vi "Summary.vi"() -> ()   [LabVIEW 2017]
uses:
  d1a68c5a-fde4-43d3-b03d-75d6c03e9ac0.vi
  12295e0e-d0dd-4d64-ad21-811591a871be.vi
panel:
  out "Value 2":i32
  out "Name 1":string
  out "Value 1":i32
  out "Name 2":string
  # "Summary Points:\n  - VIMs are more flexible than Polymorphic VIs\n  - They are easier to write than XNodes\n  - At some undefined point in the future, they will be available in NXG\n  - VIMs cannot be the top level entry in a PolyVI (but they can be used in VIs that are instances of a PolyVI)  \n  - Improvements and extensions to the 'Type Algebra' system are under construction\n  - Research is ongoing at NI R&D to implement recursive VIMs\n  - There is no existing tool to convert Polymorphic VIs to VIMs\n  - In the future, classes might receive better type handling, in a 'traits-lite' style design\n  - You can place a TSS in another TSS\n  - Methods are not coerced for Property Nodes. Coercion dots do not appear outside of a VIM if coercion occurs inside the VIM. Clusters can be unbundled by name even if they are not of the same type"
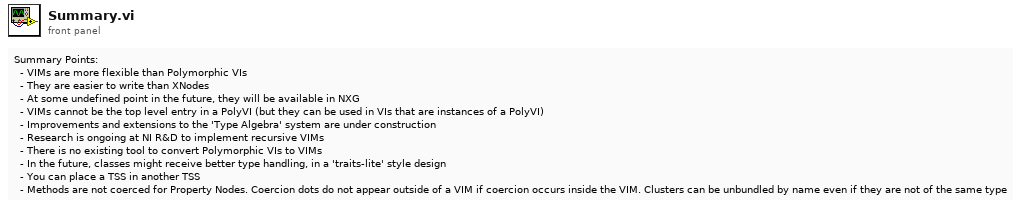
[diagram p1: front panel]
types:
  T1 = cluster{"Value":i32, "Type":enum16{"Type A", "Type B"}, "Boolean":bool, "Odd":string}
  T2 = cluster{"Name":string, "Value":i32, "Type":enum16{"Type A", "Type B"}}
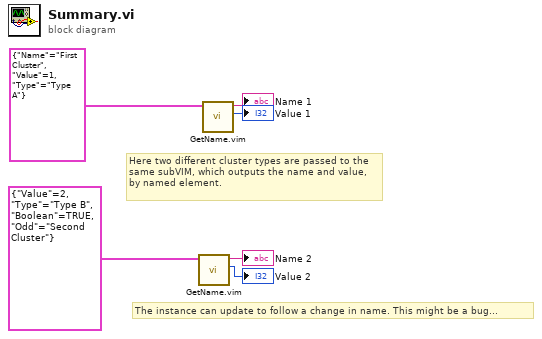
[diagram p0: block diagram]
diagram:
  # "The instance can update to follow a change in name. This might be a bug..."
  # "Here two different cluster types are passed to the same subVIM, which outputs the name and value, by named element."
  n1 = call "GetName.vim"("Cluster"=T1 {"Value"=2, "Type"=enum."Type B", "Boolean"=TRUE, "Odd"="Second Cluster"}) -> ("Value"=→"Value 2":i32, "Name"=→"Name 2":string)  [unwired: 9 in]
  n2 = call "GetName.vim"("Cluster"=T2 {"Name"="First Cluster", "Value"=1, "Type"=enum."Type A"}) -> ("Value"=→"Value 1":i32, "Name"=→"Name 1":string)  [unwired: 9 in]
